vi "to_table.vi"(8 "error in (no error)":errorcluster, 11 "Item in":refnum<class "Item.lvclass">) -> (0 "error out":errorcluster, 3 "Table":refnum<class "Table.lvclass">)   [LabVIEW 2020, in "toml_edit.lvlib" / "Item.lvclass"]
uses:
  Item.lvclass
  Table/Table.lvclass
  Item.lvclass/Item.ctl
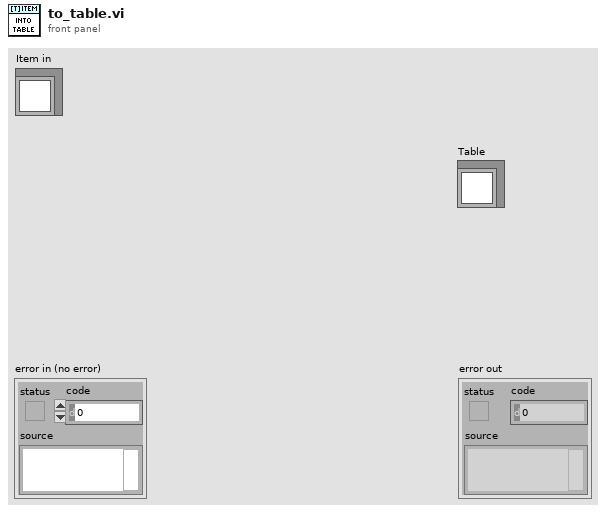
[diagram p1: front panel]
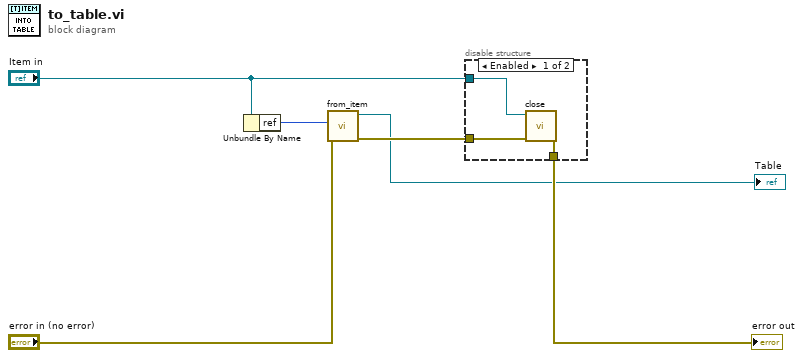
[diagram p0: block diagram]
diagram:
  n1 = Unbundle By Name("Item in") -> ("ref"=w6:u64)
  n2 = call "from_item.vi"("error in (no error)"="error in (no error)", "item_ref"=w6) -> ("error out"=w5:errorcluster, "Table out"=→"Table":refnum<class "Table.lvclass">)  [unwired: 8 in]
  n3 = disable-structure shown="Enabled" {
    disable-tunnel: w5 -> [w9 w10]
    disable-tunnel: [w8 w10] -> w4
    disable-tunnel: "Item in" -> [w7 _]
    frame Enabled {
      n4 = call "close.vi"("error in (no error)"=w9, "Item in"=w7) -> ("error out"=w8:errorcluster)  [unwired: 9 in]
    }
    frame Disabled {
    }
  }
  "error out" <- w4
